vi "ADXRS453_Read.vi"(8 "Error In":errorcluster, 10 "Gyro Detected?":bool, 11 "ADXRS453 Ref In":T1={"DevStatus"={"status"=FALSE, "code"=0, "source"=""}, "Handle"=0, "Controller"=enum."Controller 1", "SPI Bus"=enum."Invalid"}) -> (0 "Error Out":errorcluster, 3 "ADXRS453 Ref Out":T1={"DevStatus"={"status"=FALSE, "code"=0, "source"=""}, "Handle"=0, "Controller"=enum."Controller 1", "SPI Bus"=enum."Invalid"})   [LabVIEW 2014]
uses:
  <vilib>/Rock Robotics/WPI/SPI/WPI_SPIDevRef.ctl
  <vilib>/Rock Robotics/SystemInterfaces/Typedef/FPGA_TypedefDigitalModule.ctl
  <vilib>/Rock Robotics/SystemInterfaces/spilib/spi_bus.ctl
  <vilib>/Platform/TimedLoop/XDataNode/timing_clust.ctl
  <vilib>/Platform/TimedLoop/XDataNode/nitl_modes.ctl
  <vilib>/Platform/TimedLoop/XDataNode/wakeup.ctl
  ADXRS453_Global.vi
  <vilib>/platform/TimedLoop/XDataNode/XDataNode.xnode
  <vilib>/Platform/TimedLoop/XDataNode/XDNodeRunTimeDep.lvlib
panel:
  out "Gyro Angle":dbl
  out "Gyro Output (dps)":dbl
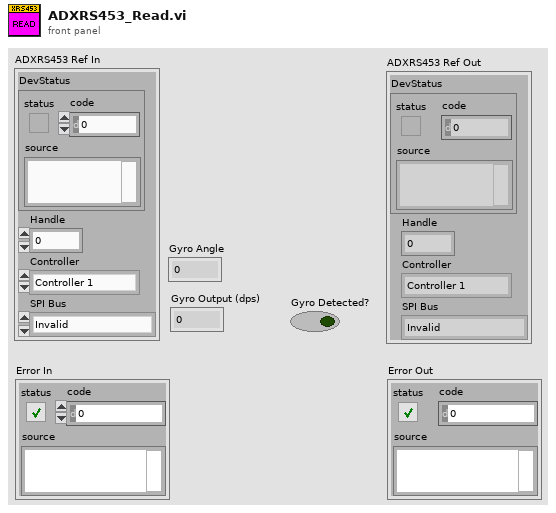
[diagram p1: front panel]
types:
  T1 = typedef "WPI_SPIDevRef.ctl" = cluster{"DevStatus":errorcluster, "Handle":i32, "Controller":T2, "SPI Bus":T3}
  T2 = typedef "FPGA_TypedefDigitalModule.ctl" = enum16{"Controller 1"}
  T3 = typedef "spi_bus.ctl" = enum16{"SPI On-Board, CS0", "SPI On-Board, CS1", "SPI On-Board, CS2", "SPI On-Board, CS3", "SPI MXP", "Invalid"}
  T4 = typedef "XDNodeRunTimeDep.lvlib/timing_clust.ctl" = cluster{"Expected End [f-1]":u64, "Actual End [f-1]":u64, "Finished Late? [f-1]":bool, "Expected End [i-1]":u64, "Actual End [i-1]":u64, "Finished Late? [i-1]":bool, "Expected Start [i]":u64, "Actual Start [i]":u64, "Expected Start [f]":u64, "Actual Start [f]":u64, "Source Name":string, "Structure Name":string, "Period":i64, "Deadline":i64, "Offset":i64, "Start":i64, "Priority":i32, "Timeout":i32, "Mode":T5, "Wakeup Reason":T6, "Error":errorcluster, "Source Type":string, "Secondary Source Type":string, "Global End Time":u64, "Global Start Time":u64, "Frame Duration":u64, "Iteration Duration":u64, "Assigned CPU":i32, "I/O Scan Engine Mode":u32}
  T5 = typedef "XDNodeRunTimeDep.lvlib/nitl_modes.ctl" = enum32{"No Change", "Process missed periods, maintain original phase", "Discard missed periods, maintain original phase", "Process missed periods, ignore original phase", "Discard missed periods, ignore original phase"}
  T6 = typedef "XDNodeRunTimeDep.lvlib/wakeup.ctl" = enum32{"Normal", "Aborted", "Asynchronous wakeup", "Timing source error", "Timed loop error", "Timeout"}
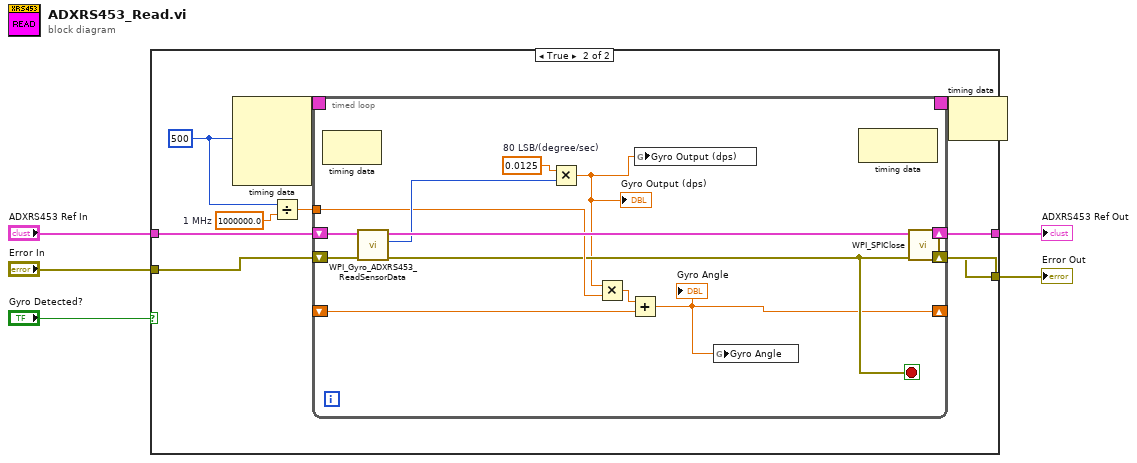
[diagram p0: block diagram]
diagram:
  n1 = case shown="True" "Gyro Detected?" {
    tunnel: "ADXRS453 Ref In" -> [w7 w14]
    tunnel: "Error In" -> [w6 w13]
    tunnel: [w6 w12] -> w5
    tunnel: [w7 w11] -> w4
    frame False {
    }
    frame True {
      w10 = 1000000.0  # 1 MHz
      w8 = i64 500 ("Period")
      n2 = node-c288(w8) -> (w16:T4)  [unwired: 3 in]
      n3 = Divide(x=w8, y=w10) -> (x/y=w9:dbl)
      n4 = timed-loop {
        shift-right: [w25] -> w11
        shift-left: w14 -> [w27]
        shift-right: [w19] -> w12
        shift-left: w13 -> [w26]
        timing: w16 -> [_]
        timing-out: [_] -> w15
        shift-right: [w17] -> _
        shift-left: _ -> [w22]
        tunnel: w9 -> [w20]
        stop <- w19 stop-if-true
        w23 = 0.0125  # 80 LSB/(degree/sec)
        n5 = node-c288() -> ()  [unwired: 1 in, 1 out]
        n6 = call <vilib>:"WPI_Gyro_ADXRS453_ReadSensorData.vi"("error in (no error)"=w26, "SPIDevRef in"=w27) -> ("error out"=w19:errorcluster, "Sensor Data (n-1)"=w24:i16, "SPIDevRef out"=w25:T1)  [unwired: 5 in, 2 out]
        n7 = Multiply(x=w23, y=w24) -> (x*y=w18:dbl)
        "Gyro Output (dps)" <- w18
        n8 = Multiply(x=w18, y=w20) -> (x*y=w21:dbl)
        n9 = Add(x=w21, y=w22) -> (x+y=w17:dbl)
        "Gyro Angle" <- w17
        n10 = global write "ADXRS453_Global.vi" "Gyro Output (dps)"(w18) -> ()
        n11 = global write "ADXRS453_Global.vi" "Gyro Angle"(w17) -> ()
        n12 = node-c288() -> ()  [unwired: 1 in, 1 out]
      }
      n13 = node-c288(w15) -> ()  [unwired: 1 out]
    }
  }
  "ADXRS453 Ref Out" <- w4
  "Error Out" <- w5
  n14 = call <vilib>:"WPI_SPIClose.vi"("error in (no error)"=w5, "SPIDevRef"=w4) -> ()  [unwired: 9 in, 1 out]
